vi "drawRoundRectangleGradientFill.vi"(0 "reference":refnum<class "Graphics.lvclass">, 1 "rectangle":T1 {"height" format="%.2f"; "width" format="%.2f"; "y" format="%.2f"; "x" format="%.2f"}, 2 "lineWidth(1)":dbl=1.0 format="%.2f", 3 "color(if not used=default color)":u32=33554432 format="%.0x", 4 "fill?(F)":bool, 5 "error in (no error)":errorcluster, 7 "RoundRadius":i16=20, 9 "TopFillColor":u32=16777216 format="%.0x", 11 "BottomFillColor":u32=16777216 format="%.0x") -> (14 "reference out":refnum<class "Graphics.lvclass">, 19 "error out":errorcluster)   [LabVIEW 2020, in "Graphics.lvclass"]
uses:
  <resource>/Framework/Providers/Open_GDS/UML/Graphics_class/Graphics.lvclass
  <resource>/Framework/Providers/Open_GDS/UML/General/Rectangle/Rectangle Rectangle2D.ctl
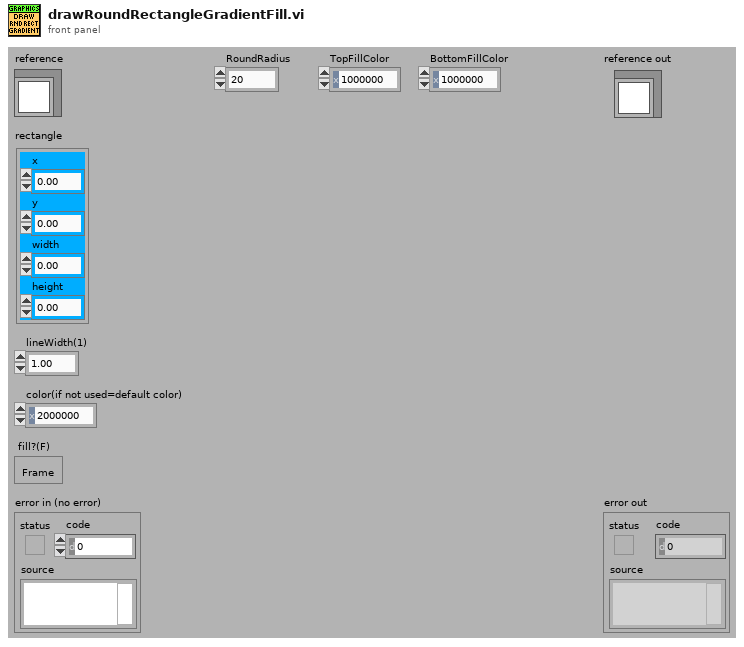
[diagram p1: front panel]
types:
  T1 = typedef "Rectangle Rectangle2D.ctl" = cluster{"x":dbl, "y":dbl, "width":dbl, "height":dbl}
  T2 = cluster{"Width":i16, "Style":enum32{"Solid", "Dash", "Dot", "DashDot", "DashDotDot"}}
  T3 = cluster{"Border":enum16{"No Border", "Rectangle", "Rounded Rectangle"}, "Border Color":u32, "Border Width":i16, "Oval Width":i16, "Oval Height":i16}
  T4 = typedef "Graphics.lvclass/ObjectAttributes.ctl" = cluster{"drawColor":u32, "backgroundColor":u32, "font":T5, "fontType":T6, "picture":picture, "stroke":T7, "scaleX":dbl, "scaleY":dbl, "screenRef":refnum<vi>, "offsetX":dbl, "offsetY":dbl}
  T5 = typedef "Graphics.lvclass/FontType.ctl" = cluster{"Font Name:":string, "Size":i16, "Strikeout?":bool, "Italic?":bool, "Underline?":bool, "Outline?":bool, "Shadow?":bool, "Bold?":bool}
  T6 = typedef "Graphics.lvclass/LvFontType.ctl" = enum16{"User-specified Font", "Application Font", "System Font", "Dialog Font"}
  T7 = typedef "Graphics.lvclass/StrokeType.ctl" = enum16{"USE_DEFAULT", "SOLID", "DOTTED"}
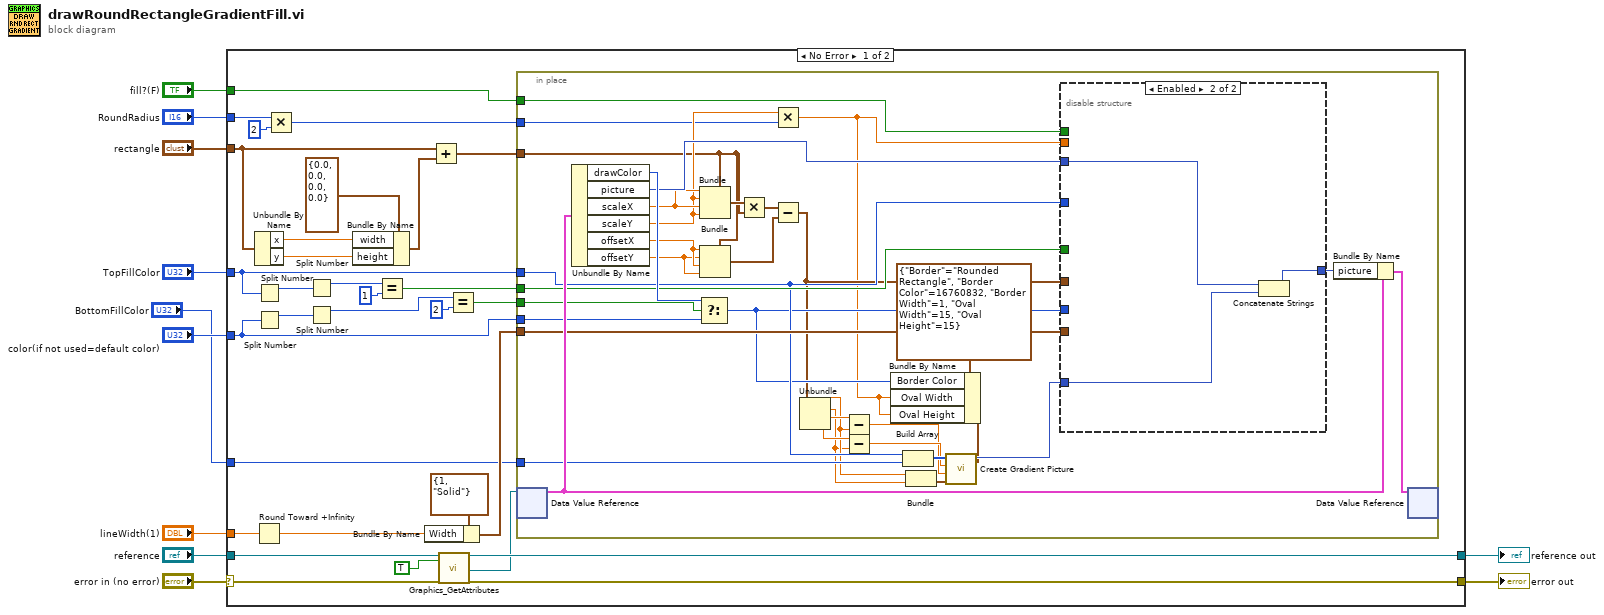
[diagram p0: block diagram]
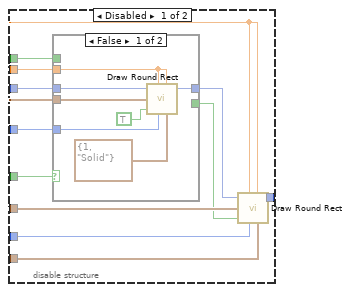
[diagram p2: hidden frame]
diagram:
  n1 = case shown="No Error" "error in (no error)" {
    selector: "error in (no error)" -> [w39 w101]
    tunnel: "reference" -> [w42 w102]
    tunnel: [w41 w101] -> w10
    tunnel: [w40 w102] -> w9
    tunnel: "rectangle" -> [w38 _]
    tunnel: "lineWidth(1)" -> [w37 _]
    tunnel: "color(if not used=default color)" -> [w19 _]
    tunnel: "fill?(F)" -> [w16 _]
    tunnel: "RoundRadius" -> [w36 _]
    tunnel: "TopFillColor" -> [w15 _]
    tunnel: "BottomFillColor" -> [w12 _]
    frame No Error {
      n2 = Round Toward +Infinity(x=w37) -> (ceil(x): smallest int >= x=w23:dbl)
      n3 = Unbundle By Name(w38) -> ("x"=w31:dbl, "y"=w30:dbl)
      n4 = Split Number(x=w15) -> (hi(x)=w25:u16)  [unwired: 1 out]
      n5 = Split Number(x=w19) -> (hi(x)=w35:u16)  [unwired: 1 out]
      n6 = Multiply(x=w36, y=i16 2) -> (x*y=w14:i16)
      n7 = Split Number(x=w25) -> (hi(x)=w26:u8)  [unwired: 1 out]
      n8 = Split Number(x=w35) -> (hi(x)=w34:u8)  [unwired: 1 out]
      n9 = Bundle By Name(cluster=T1 {"x"=0.0, "y"=0.0, "width"=0.0, "height"=0.0} ("x"), "width"=w31, "height"=w30) -> (w29:T1)
      n10 = Equal?(x=w26, y=u8 1) -> (x = y?=w17:bool)
      n11 = Bundle By Name(cluster=T2 {"Width"=1, "Style"=enum."Solid"} ("pen"), "Width"=w23) -> (w20:T2)
      n12 = Add(x=w38, y=w29) -> (x+y=w13:T1)
      n13 = call <resource>:"Graphics_GetAttributes.vi"("reference in"=w42, "OnlyGetDvrReference(False)"=TRUE, "error in (no error)"=w39) -> ("reference out"=w40:refnum<class "Graphics.lvclass">, "DataRef"=w21:refnum<data-value>, "error out"=w41:errorcluster)  [unwired: 13 in, 1 out]
      n14 = Equal?(x=w34, y=u8 2) -> (x = y?=w18:bool)
      n15 = in-place {
        in-place-border: w20 -> [w68]
        in-place-border: w19 -> [w67]
        in-place-border: w18 -> [w66]
        in-place-border: w17 -> [w65]
        in-place-border: w16 -> [w64]
        in-place-border: w15 -> [w58]
        in-place-border: w14 -> [w62]
        in-place-border: w13 -> [w59]
        in-place-border: w12 -> [w57]
        n16 = in-place-dvr #1(w21) -> (w77:T4)  [unwired: 1 out]
        n17 = Unbundle By Name(w77) -> ("drawColor"=w74:u32, "picture"=w73:picture, "scaleX"=w72:dbl, "scaleY"=w71:dbl, "offsetX"=w70:dbl, "offsetY"=w69:dbl)
        n18 = Select(t=w74, s=w66, f=w67) -> (s? t:f=w52:u32)
        n19 = Bundle(cluster=w59, "x"=w72, "y"=w71, "width"=w72, "height"=w71) -> (w63:T1)
        n20 = Bundle(cluster=w59, "x"=w70, "y"=w69, "width"=w70, "height"=w69) -> (w61:T1)
        n21 = Multiply(x=w63, y=w59) -> (x*y=w60:T1)
        n22 = Multiply(x=w71, y=w62) -> (x*y=w43:dbl)
        n23 = Subtract(x=w60, y=w61) -> (x-y=w51:T1)
        n24 = Unbundle(w51) -> ("x"=w48:dbl, "y"=w47:dbl, "width"=w50:dbl, "height"=w49:dbl)
        n25 = Subtract(x=w50, y=w48) -> (x-y=w44:dbl)
        n26 = Subtract(x=w49, y=w47) -> (x-y=w45:dbl)
        n27 = Bundle By Name(cluster=T3 {"Border"=enum."Rounded Rectangle", "Border Color"=16760832, "Border Width"=1, "Oval Width"=15, "Oval Height"=15} ("Border Settings"), "Border Color"=w52, "Oval Width"=w43, "Oval Height"=w43) -> (w53:T3)
        n28 = Build Array(w58, w57) -> (w56:u32[])
        n29 = Bundle("x"=w48, "y"=w47) -> (w46:cluster{"x":dbl, "y":dbl})  [unwired: 1 in]
        n30 = call <resource>:"Create Gradient Picture.vi"("Border Settings"=w53, "Offset"=w46, "Width"=w44, "Height"=w45, "Color Array"=w56) -> ("Gradient Picture"=w55:picture)  [unwired: 6 in]
        n31 = disable-structure shown="Enabled" {
          disable-tunnel: [w88 w98] -> w76
          disable-tunnel: w73 -> [w87 w100]
          disable-tunnel: w43 -> [w85 _]
          disable-tunnel: w51 -> [w84 _]
          disable-tunnel: w52 -> [w82 _]
          disable-tunnel: w68 -> [w81 _]
          disable-tunnel: w65 -> [w80 _]
          disable-tunnel: w64 -> [w79 _]
          disable-tunnel: w58 -> [w78 _]
          disable-tunnel: w55 -> [_ w99]
          frame Disabled {
            n32 = case shown="False" w80 {
              tunnel: w79 -> [_ w97]
              tunnel: [_ w97] -> w83
              tunnel: w87 -> [w95 w96]
              tunnel: [w94 w96] -> w86
              tunnel: w78 -> [w92 _]
              tunnel: w85 -> [w93 _]
              tunnel: w84 -> [w90 _]
              frame False {
                n33 = call <vilib>:"Draw Round Rect.vi"("picture"=w95, "oval width"=w93, "rect"=w90, "fill?(F)"=TRUE, "color(black)"=w92, "oval height"=w93, "pen"=T2 {"Width"=1, "Style"=enum."Solid"}) -> ("new picture"=w94:picture)  [unwired: 2 out]
              }
              frame True {
              }
            }
            n34 = call <vilib>:"Draw Round Rect.vi"("picture"=w86, "oval width"=w85, "rect"=w84, "fill?(F)"=w83, "color(black)"=w82, "oval height"=w85, "pen"=w81) -> ("new picture"=w88:picture)  [unwired: 2 out]
          }
          frame Enabled {
            n35 = Concatenate Strings(w100, w99) -> (w98:picture)
          }
        }
        n36 = Bundle By Name(cluster=w77, "picture"=w76) -> (w75:T4)
        n37 = in-place-dvr #1(w75) -> ()  [unwired: 2 out]
      }
    }
    frame Error {
    }
  }
  "reference out" <- w9
  "error out" <- w10
